vi "Stop Core.vi"(10 "final error code":i32, 11 "Hardware Buzzer in":refnum<class "Hardware Buzzer.lvclass">) -> (3 "Hardware Buzzer out":refnum<class "Hardware Buzzer.lvclass">)   [LabVIEW 2021, in "Hardware Buzzer.lvlib" / "Hardware Buzzer.lvclass"]
doc: "<p>(<strong>Filename</strong>: <span class=\"dnl\">Actor Framework.lvlib:Actor.lvclass:Stop Core.vi</span>)</p>\n<p>Defines what the actor does before it stops. Use the <strong>final error code</strong> input to determine whether the actor shut down in response to an error.</p>\n<p>By default, this method passes the Stop message along to all <a href=\"nihelplauncher://docs/csh?context=lvcore_lvcomm_af_launch_nested_actor\">auto-stop nested actors</a>. A descendant class may override this method to define additional behavior, such as shutting down any processes the actor initiated in its override of the <a href=\"nihelplauncher://docs/csh?context=lvcore_lvcomm_af_actor_core\">Actor Core</a> method.</p>"
uses:
  Hardware Buzzer.lvclass
  Hardware Buzzer.lvclass/Hardware Buzzer.ctl
  <vilib>/ActorFramework/Actor/Actor.lvclass
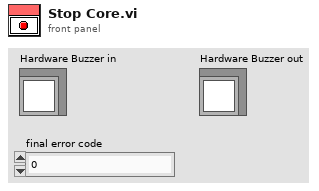
[diagram p1: front panel]
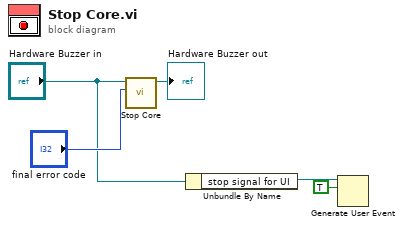
[diagram p0: block diagram]
diagram:
  n1 = call-parent "Stop Core.vi"("final error code"="final error code", "Actor in"="Hardware Buzzer in") -> ("Actor out"=→"Hardware Buzzer out":refnum<class "Hardware Buzzer.lvclass">)  [unwired: 9 in]
  n2 = Unbundle By Name("Hardware Buzzer in") -> ("stop signal for UI"=w3:refnum<user-event>)
  n3 = Generate User Event(user event=w3, event data cluster=TRUE ("event data")) -> ()  [unwired: 2 in, 2 out]
